vi "Write.vi"(8 "error in (no error)":errorcluster, 9 "Timeout S (0)":dbl, 10 "Data":string, 11 "VisaResource in":refnum<class "VisaResource.lvclass">) -> (0 "error out":errorcluster, 2 "Bytes Written":i32, 3 "VisaResource out":refnum<class "VisaResource.lvclass">)   [LabVIEW 2020, in "PicoG-Core.lvlib" / "VisaResource.lvclass"]
uses:
  VisaResource.lvclass
  VisaResource.lvclass/VisaResource.ctl
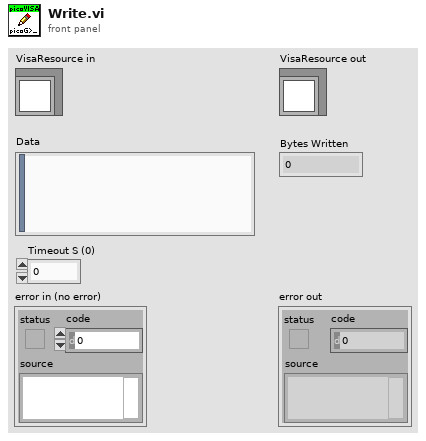
[diagram p1: front panel]
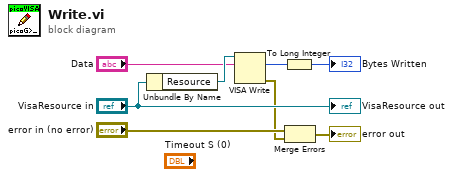
[diagram p0: block diagram]
diagram:
  n1 = Unbundle By Name("VisaResource in") -> ("Resource"=w6:refnum<visa-resource-name>)
  n2 = VISA Write(VISA resource name=w6, write buffer="Data") -> (return count=w4:u32, error out=w1:errorcluster)  [unwired: 1 in, 1 out]
  n3 = To Long Integer(number=w4) -> (32bit integer=→"Bytes Written":i32)
  n4 = Merge Errors("error in (no error)", w1) -> (→"error out":errorcluster)
  "VisaResource out" <- "VisaResource in"
